vi "STM Basic Client Example.vi"() -> ()   [LabVIEW 2010]
doc: "This example demonstrates how to implement a STM client which receives messages from the server.\n\nThe server needs to be started before the client."
uses:
  vi.lib/NI/STM/TCP/Read Meta Data (TCP Ref).vi
  vi.lib/NI/STM/TCP/Get Connection Reference (TCP).vi
  vi.lib/NI/STM/TCP/Read Meta Data (TCP Clst).vi
  vi.lib/NI/STM/TCP/Read Message (TCP).vi
  vi.lib/NI/STM/NI STM.lvlib
panel:
  out "error  out":errorcluster
  out "Data":dbl[](array[numeric])
  out "Iteration Counter":i32
  in  "Target IP Address":string="localhost"
  in  "stop":bool
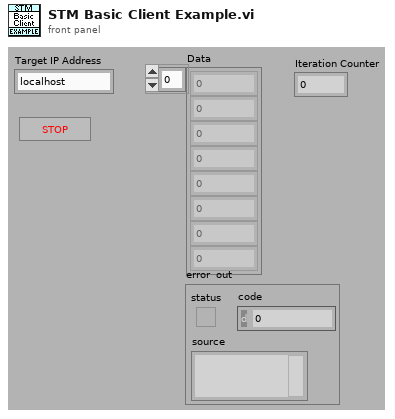
[diagram p1: front panel]
types:
  T1 = typedef "NI STM.lvlib/TCP Connection Info.ctl" = cluster{"connection ID":refnum<k5>, "meta data":T2[]}
  T2 = typedef "NI STM.lvlib/MetaDataElement.ctl" = string
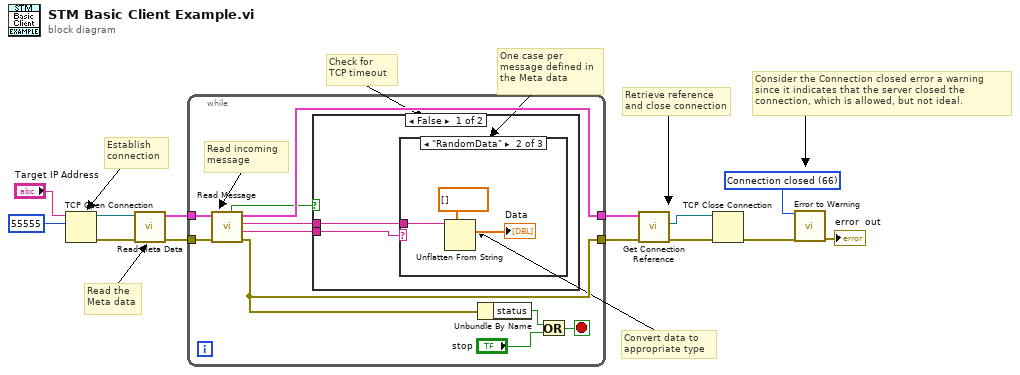
[diagram p0: block diagram]
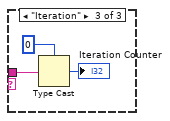
[diagram p3: hidden frame]
diagram:
  w7 = 66 items=["No Error", "Argument Error", "Memory Full", "Out of Zone", "End of File", "File Already Open", "Generic File IO Error", "File Not Found", "File Permission Error", "Disk Full", "Duplicate Path", "Too Many Files Open", "Not Enabled", "Resource File Not Found", "Cannot Add Resource", "Resource Not Found", "Image Not Found", "Image Memory Error", "Pen Does Not Exist", "Config Bad Type", "Config Token Not Found", "Config Parse Error", "Config Memory Error", "Bad External Code Format", "Bad External Code Offset", "External Code Not Present", "Null Window", "Destroy Window Mixup", "Null Menu", "Print Aborted", "Bad Print Record", "Print Driver Error", "Windows Error During Print", "Memory Error During Print", "Print Dialog Error", "Generic Print Error", "Invalid Device Refnum", "Device Not Found", "Device Parameter Error", "Device Unit Error", "Can't Open Device", "Device Call Aborted", "Generic Error", "Cancelled By User", "Object ID Too Low", "Object ID Too High", "Object Not In Heap", "Unknown Heap", "Bad DefProc ID", "DefProc Not In Table", "Message Out Of Range", "Null Method", "Unknown Message", "Manager Call Not Supported", "Bad address", "Connection In progress", "Connection timed out", "Connection is already in progress", "Network attribute not supported", "Network error", "Address in use", "System out of memory", "Connection aborted", "Connection refused", "Connection is not connected", "Connection is already connected", "Connection closed", "Initialize error (interapplication manager)", "Bad occurrence", "Wait on unbound occurrence handler", "Occurrence queue overflow", "Bad path", "Semaphore not signaled", "Unrecognized type (interapplication manager)"] ("1st Error to Convert")
  # "Consider the Connection closed error a warning since it indicates that the server closed the connection, which is allowed, but not ideal."
  # "Retrieve reference and close connection"
  # "Check for\nTCP timeout"
  # "Convert data to\nappropriate type"
  # "One case per\nmessage defined in\nthe Meta data"
  # "Read the \nMeta data"
  # "Establish\nconnection"
  n1 = TCP Open Connection(address="Target IP Address", remote port or service name=u16 55555 ("remote port")) -> (connection ID=w13:refnum<k5>, error out=w11:errorcluster)  [unwired: 1 in, 2 out]
  n2 = call-poly "Read Meta Data.vi"("error in"=w11, "connection ID"=w13) -> ("error out"=w10:errorcluster, "connection info out"=w12:T1)  [unwired: 1 in, 7 out]
  n3 = while {
    tunnel: w12 -> [w23]
    tunnel: w10 -> [w22]
    tunnel: [w21] -> w4
    tunnel: [w18] -> w3
    stop <- w15 stop-if-true
    # "Read incoming\nmessage"
    n4 = call-poly "Read Message.vi"("error in"=w22, "connection info in"=w23) -> ("error out"=w18:errorcluster, "name"=w20:T2, "data string"=w19:string, "connection info out"=w21:T1, "timed out?"=w14:bool)  [unwired: 1 in, 4 out]
    n5 = case shown="False" w14 {
      tunnel: w20 -> [w24 _]
      tunnel: w19 -> [w25 _]
      frame False {
        n6 = case shown="\"RandomData\"" w24 {
          tunnel: w25 -> [_ w28 w31]
          frame Default {
          }
          frame "RandomData" {
            n7 = Unflatten From String(type=dbl[] [], binary string=w28) -> (value=→"Data":dbl[])  [unwired: 1 in, 4 out]
          }
          frame "Iteration" {
            n8 = Type Cast(type=0, x=w31) -> (*(type *) &x=→"Iteration Counter":i32)
          }
        }
      }
      frame True {
      }
    }
    n9 = Unbundle By Name(w18) -> ("status"=w17:bool)
    n10 = Or(x=w17, y="stop") -> (x .or. y?=w15:bool)
  }
  n11 = call-poly "Get Connection Reference.vi"("error in"=w3, "connection info in"=w4) -> ("error out"=w1:errorcluster, "connection ID out"=w2:refnum<k5>)  [unwired: 8 out]
  n12 = TCP Close Connection(connection ID=w2, error in (no error)=w1) -> (error out=w6:errorcluster)  [unwired: 2 out]
  n13 = call <vilib>:"Error to Warning.vi"("1st Error to Convert"=w7, "error in"=w6) -> ("warning out"=→"error  out":errorcluster)  [unwired: 3 in, 10 out]
